vi "UDP接收.vi"(8 "匹配帧信息_异常":u16[](array[numeric]), 9 "长度":u16, 10 "匹配帧信息_正常":u16[](array[numeric])) -> (0 "异常_找到?":bool, 1 "接收超时?":bool, 2 "接收的一帧数据":u16[](array[numeric]), 3 "正常_找到?":bool)   [LabVIEW 2010]
uses:
  全局量/全局_配置.vi
panel:
  out "开始时间":dbl format="%#.0f"
  # "0:发送方标识\n1:报文类型\n2:数据区字长"
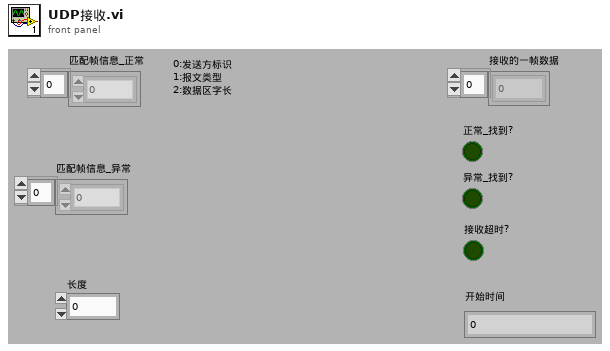
[diagram p1: front panel]
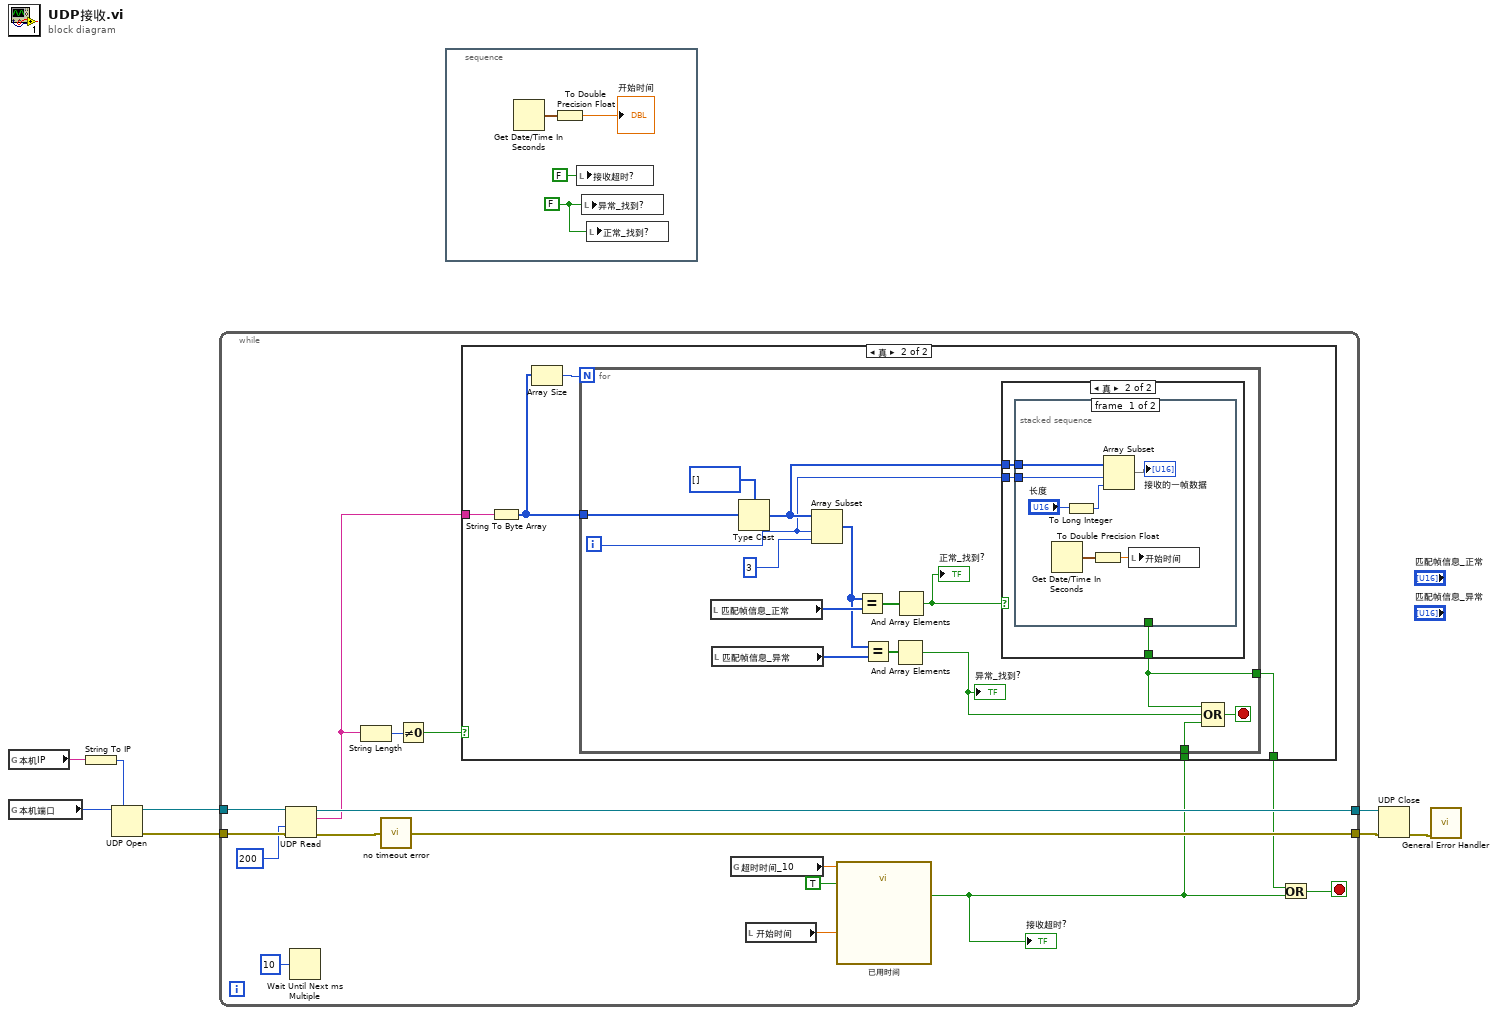
[diagram p0: block diagram]
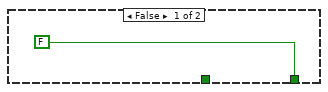
[diagram p2: hidden frame]
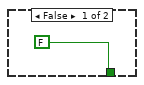
[diagram p3: hidden frame]
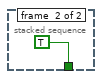
[diagram p4: hidden frame]
diagram:
  n1 = global read "全局_配置.vi" "本机IP"() -> (w3:string)
  n2 = global read "全局_配置.vi" "本机端口"() -> (w1:u16)
  n3 = String To IP(1:w3) -> (0:w2:u32)
  n4 = UDP Open(7:w2, 11:w1) -> (port=w8:refnum<k16>, 0:w7:errorcluster)  [unwired: 3 in, 1 out]
  n5 = while {
    tunnel: w8 -> [w24]
    tunnel: w7 -> [w23]
    tunnel: [w22] -> w5
    tunnel: [w21] -> w4
    stop <- w12 stop-if-true
    n6 = UDP Read(connection ID=w24, timeout ms (25000)=200, 8:w23) -> (data out=w11:string, error out=w17:errorcluster, 3:w22:refnum<k16>)  [unwired: 1 in, 2 out]
    n7 = Wait Until Next ms Multiple(millisecond multiple=u32 10 ("毫秒倍数")) -> ()  [unwired: 1 out]
    n8 = String Length(string=w11) -> (length=w19:i32)
    n9 = call "no timeout error.vi"("error in (no error)"=w17) -> ("error out"=w21:errorcluster)
    n10 = Not Equal To 0?(x=w19) -> (x != 0?=w18:bool)
    n11 = global read "全局_配置.vi" "超时时间_10"() -> (w15:dbl)
    n12 = local read "开始时间"() -> (w14:dbl)
    n13 = call "已用时间"("Time Target (s)"=w15, "Reset"=TRUE, "Set Start Time (s)"=w14) -> ("Time has Elapsed"=w9:bool)  [unwired: 9 in, 7 out]
    "接收超时?" <- w9
    n14 = case shown="真" w18 {
      tunnel: w11 -> [_ w29]
      tunnel: [FALSE ("找到?") w30] -> w13
      tunnel: w9 -> [_ w28]
      frame False {
      }
      frame True {
        n15 = String To Byte Array(string=w29) -> (unsigned byte array=w27:u8[])
        n16 = Array Size(array=w27) -> (size(s)=w26:i32)
        n17 = for {
          N: w26 -> [_]
          tunnel: w27 -> [w45]
          tunnel: [w33] -> w30
          tunnel: w28 -> [w32]
          i -> [w34]
          stop <- w35 stop-if-true
          n18 = local read "匹配帧信息_正常"() -> (w39:u16[])
          n19 = local read "匹配帧信息_异常"() -> (w41:u16[])
          n20 = Type Cast(type=u16[] [], x=w45) -> (*(type *) &x=w37:u16[])
          n21 = Array Subset(array=w37, index=w34, length=3 ("长度")) -> (w38:u16[])
          n22 = Equal?(x=w38, y=w39) -> (x = y?=w40:bool[])
          n23 = Equal?(x=w38, y=w41) -> (x = y?=w42:bool[])
          n24 = And Array Elements(Boolean array=w42) -> (logical AND=w31:bool)
          "异常_找到?" <- w31
          n25 = And Array Elements(Boolean array=w40) -> (logical AND=w36:bool)
          "正常_找到?" <- w36
          n26 = case shown="真" w36 {
            tunnel: [FALSE w47] -> w33
            tunnel: w37 -> [_ w49]
            tunnel: w34 -> [_ w48]
            frame False {
            }
            frame True {
              n27 = stacked-sequence {
                tunnel: w49 -> [w56 _]
                tunnel: w48 -> [w55 _]
                tunnel: [_ TRUE] -> w47
                frame #0 {
                  n28 = Get Date/Time In Seconds() -> (seconds since 1Jan1904=w52:timestamp)
                  n29 = To Long Integer(number="长度") -> (32bit integer=w53:i32)
                  n30 = To Double Precision Float(number=w52) -> (double precision float=w51:dbl)
                  n31 = Array Subset(array=w56, index=w55, length=w53) -> (→"接收的一帧数据":u16[])
                  n32 = local write "开始时间"(w51) -> ()
                }
                frame #1 {
                }
              }
            }
          }
          n33 = Compound Arithmetic op=OR(w33, w31, w32) -> (w35:bool)
        }
      }
    }
    n34 = Or(x=w13, y=w9) -> (x .or. y?=w12:bool)
  }
  n35 = stacked-sequence {
    frame #0 {
      w59 = FALSE ("找到?")
      n36 = Get Date/Time In Seconds() -> (seconds since 1Jan1904=w61:timestamp)
      n37 = To Double Precision Float(number=w61) -> (double precision float=→"开始时间":dbl)
      n38 = local write "接收超时?"(FALSE ("接收超时?")) -> ()
      n39 = local write "异常_找到?"(w59) -> ()
      n40 = local write "正常_找到?"(w59) -> ()
    }
  }
  n41 = UDP Close(connection ID=w5, 8:w4) -> (error out=w6:errorcluster)  [unwired: 1 out]
  n42 = call <vilib>:"General Error Handler.vi"("error in (no error)"=w6) -> ()  [unwired: 10 in, 5 out]
